vi "DHE_GetFromDBS.vi"(8 "error in (no error)":errorcluster, 11 "Database RefNum in":T1) -> (0 "error out":errorcluster, 1 "coadds":i32, 2 "fsamples":i32, 3 "exptime":i32, 4 "nimages":i32, 5 "readtime":i32, 6 "sur":i32, 7 "image_factor":i32)   [LabVIEW 2016]
uses:
  DBSHAND/private/vis/DatabaseHand_RefNum.ctl
  DBSHAND/private/vis/DatabaseHand_Element_Get(double).vi
  DBSHAND/private/vis/DatabaseHand_Element_Get(I32).vi
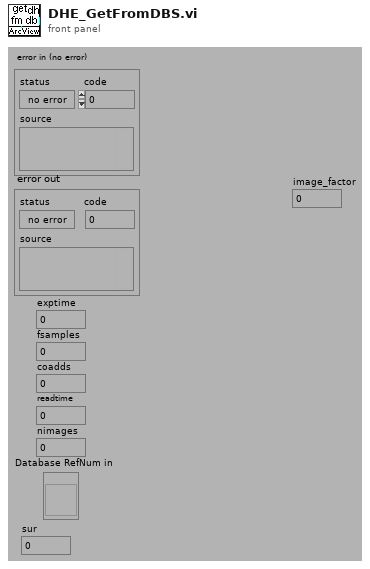
[diagram p1: front panel]
types:
  T1 = typedef "DatabaseHand_RefNum.ctl" = refnum<vi>
  T2 = cluster{"Video Processor Type":string, "support gain":bool, "Timing Board":string, "support reset":bool, "Utility Board":string, "Shutter":string, "Temperature":string, "support temp control":bool, "Detector Type":string, "Support MPP":string, "Support Binning":string, "Readout Mode":string, "support shutter control":bool}
  T3 = typedef "CMN_ContStatus.ctl" = cluster{"Response":string, "power":bool, "shutter":bool, "artifdata":bool, "idlemode":bool, "reset":bool, "gain":u8, "speed":u8, "resetPCI":bool, "autoshutter":bool, "TempSetPoint":i32, "multipleextensions":bool, "displayImage":bool, "coadding":bool, "images being coadded":i32, "Operation Mode":enum16{"normal", "coadd", "fawler"}, "frames to write":cluster{"subs":bool, "reset":bool, "exposed":bool}, "fawler samples":i32, "write auto":bool, "datatype":string, "frames to display":cluster{"subs":bool, "reset":bool, "exposed":bool}, "sur":i32, "autoclear":bool}
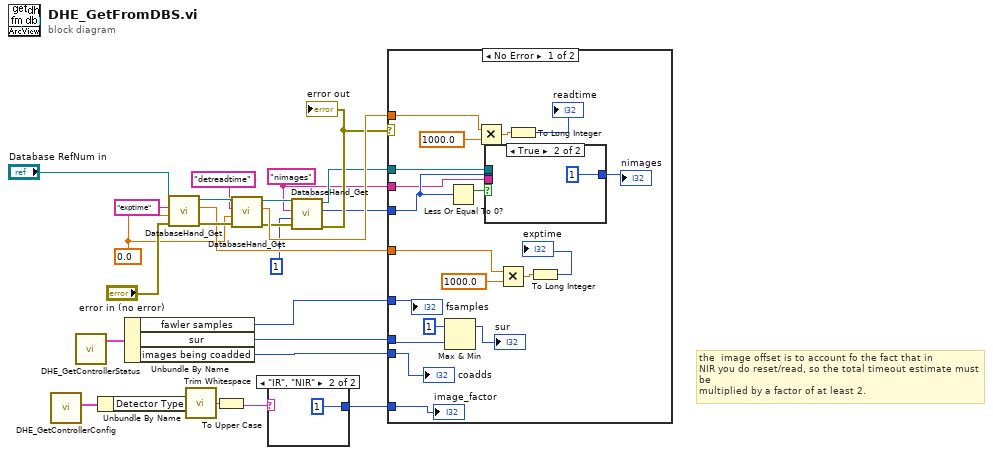
[diagram p0: block diagram]
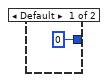
[diagram p2: hidden frame]
diagram:
  w8 = "nimages" ("name")
  w18 = 0.0
  # "the  image offset is to account fo the fact that in\nNIR you do reset/read, so the total timeout estimate must be\nmultiplied by a factor of at least 2."
  n1 = call "DHE_GetControllerConfig.vi"() -> ("ControllerConfigCluster"=w6:T2)  [unwired: 11 out]
  n2 = call "DHE_GetControllerStatus.vi"() -> ("ControllerStatus"=w25:T3)  [unwired: 11 out]
  n3 = Unbundle By Name(w6) -> ("Detector Type"=w5:string)
  n4 = Unbundle By Name(w25) -> ("fawler samples"=w11:i32, "sur"=w3:i32, "images being coadded"=w10:i32)
  n5 = call-poly "DatabaseHand_Get.vi"("error in (no error)"="error in (no error)", "default value"=w18, "name"="exptime", "Database RefNum in"="Database RefNum in") -> ("error out"=w20:errorcluster, "value"=w19:dbl, "Database RefNum out"=w23:T1)  [unwired: 1 in, 4 out]
  n6 = call <vilib>:"Trim Whitespace.vi"("string"=w5) -> ("trimmed string"=w4:string)  [unwired: 1 in]
  n7 = To Upper Case(1:w4) -> (0:w2:string)
  n8 = call-poly "DatabaseHand_Get.vi"("error in (no error)"=w20, "default value"=w18, "name"="detreadtime", "Database RefNum in"=w23) -> ("error out"=w16:errorcluster, "value"=w17:dbl, "Database RefNum out"=w15:T1)  [unwired: 1 in, 4 out]
  n9 = case shown="\"IR\", \"NIR\"" w2 {
    tunnel: [0 ("factor") 1 ("factor")] -> w1
    frame Default {
    }
    frame "IR", "NIR" {
    }
  }
  n10 = call-poly "DatabaseHand_Get.vi"("error in (no error)"=w16, "default value"=1, "name"=w8, "Database RefNum in"=w15) -> ("error out"=w13:errorcluster, "value"=w12:i32, "Database RefNum out"=w9:T1)  [unwired: 1 in, 4 out]
  "error out" <- w13
  n11 = case shown="No Error" w13 {
    tunnel: w19 -> [w40 _]
    tunnel: w17 -> [w39 _]
    tunnel: w12 -> [w35 _]
    tunnel: w11 -> [w38 _]
    tunnel: w3 -> [w30 _]
    tunnel: w10 -> [w37 _]
    tunnel: w9 -> [w33 _]
    tunnel: w8 -> [w32 _]
    tunnel: w1 -> [w31 _]
    frame No Error {
      n12 = Max & Min(x=1, y=w30) -> (max(x,y)=→"sur":i32)  [unwired: 1 out]
      n13 = Less Or Equal To 0?(x=w35) -> (x <= 0?=w36:bool)
      n14 = Multiply(x=w39, y=1000.0) -> (x*y=w43:dbl)
      n15 = case shown="True" w36 {
        tunnel: w35 -> [w47 _]
        tunnel: [w47 1 ("value")] -> w34
        tunnel: w33 -> [_ _]
        tunnel: w32 -> [_ _]
        frame False {
        }
        frame True {
        }
      }
      "nimages" <- w34
      n16 = Multiply(x=w40, y=1000.0) -> (x*y=w45:dbl)
      n17 = To Long Integer(number=w43) -> (32bit integer=→"readtime":i32)
      n18 = To Long Integer(number=w45) -> (32bit integer=→"exptime":i32)
      "fsamples" <- w38
      "coadds" <- w37
      "image_factor" <- w31
    }
    frame Error {
    }
  }
